vi "PCO_Grab_Save.vi"(7 "# of frames":u16, 8 "entrée d'erreur (pas d'erreur)":errorcluster, 9 "Message Data":variant, 11 "Camera en entrée":refnum<class "Camera.lvclass">) -> (0 "sortie d'erreur":errorcluster, 1 "meta_data_list":T1(array[cluster]), 2 "Raw data (U16)":u16[][][](array[numeric]), 3 "Camera en sortie":refnum<class "Camera.lvclass">)   [LabVIEW 2026]
uses:
  <instrlib>/PCO_SDK/File Group 0/vi.lib/Excelitas PCO GmbH/pco.labview/camera/Camera.lvclass
  Controls/PCO_Config.ctl
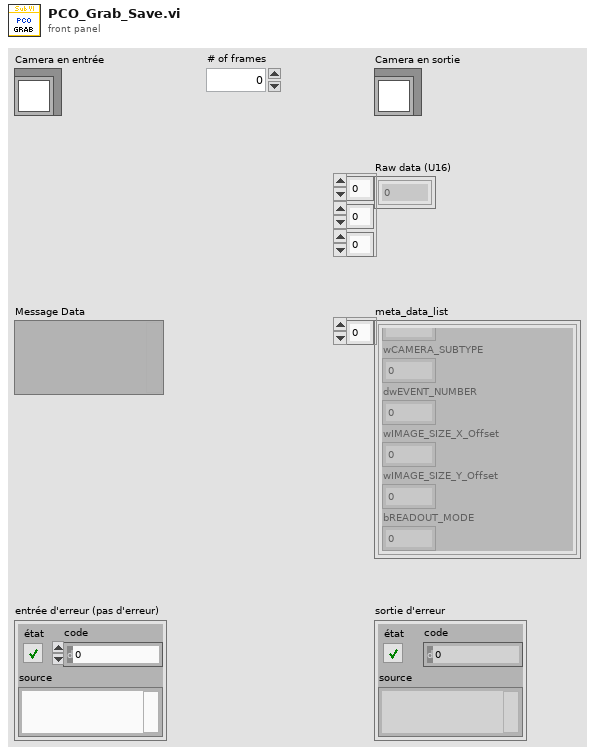
[diagram p1: front panel]
types:
  T1 = cluster{"wVersion":u16, "dwIMAGE_COUNTER":u32, "dwIMAGE_TIME_US":u32, "lvTimestamp":timestamp, "bIMAGE_TIME_STATUS":u8, "wEXPOSURE_TIME_BASE":u16, "dwEXPOSURE_TIME":u32, "dwFRAMERATE_MILLIHZ":u32, "sSENSOR_TEMPERATURE":i16, "wIMAGE_SIZE_X":u16, "wIMAGE_SIZE_Y":u16, "bBINNING_X":u8, "bBINNING_Y":u8, "dwSENSOR_READOUT_FREQUENCY":u32, "wSENSOR_CONV_FACTOR":u16, "dwCAMERA_SERIAL_NO":u32, "wCAMERA_TYPE":u16, "bBIT_RESOLUTION":u8, "bSYNC_STATUS":u8, "wDARK_OFFSET":u16, "bTRIGGER_MODE":u8, "bDOUBLE_IMAGE_MODE":u8, "bCAMERA_SYNC_MODE":u8, "bIMAGE_TYPE":u8, "wCOLOR_PATTERN":u16, "wCAMERA_SUBTYPE":u16, "dwEVENT_NUMBER":u32, "wIMAGE_SIZE_X_Offset":u16, "wIMAGE_SIZE_Y_Offset":u16, "bREADOUT_MODE":u8}[]
  T2 = enum16{"Undefined", "Mono8", "Mono16", "BGRA8", "RGBA8", "BGRA16", "RGBA16", "CompressedMono8"}
  T3 = typedef "PCO_Config.ctl" = cluster{"Exposure time (s)":dbl, "TriggerMode":u16, "ROI X0":u16, "ROI Y0":u16, "ROI X1":u16, "ROI Y1":u16, "Binning":u8}
  T4 = enum16{"sequence", "sequence non blocking", "ring buffer", "fifo", "sequence_dpcore", "sequence_non_blocking_dpcore", "ring_buffer_dpcore", "fifo_dpcore", "tif", "multitif", "pcoraw", "b16", "dicom", "multidicom", "camram_ring", "camram_segment"}
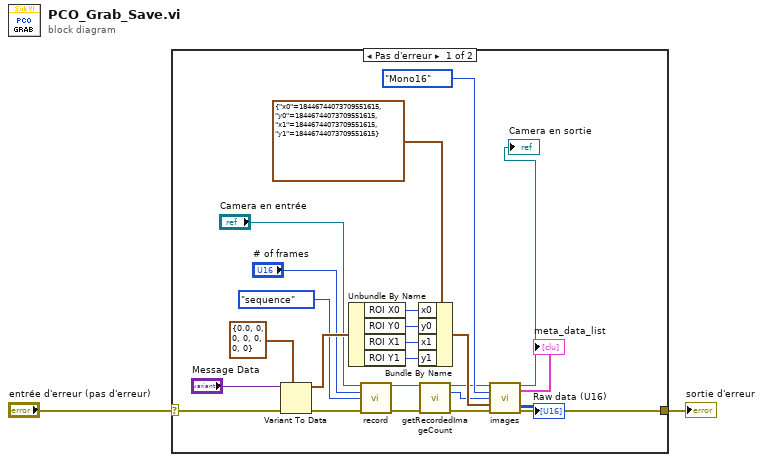
[diagram p0: block diagram]
diagram:
  n1 = case shown="Pas d'erreur" "entrée d'erreur (pas d'erreur)" {
    selector: "entrée d'erreur (pas d'erreur)" -> [w6 w27]
    tunnel: [w5 w27] -> w2
    frame No Error {
      n2 = Variant To Data(error in=w6, type=T3 {"Exposure time (s)"=0.0, "TriggerMode"=0, "ROI X0"=0, "ROI Y0"=0, "ROI X1"=0, "ROI Y1"=0, "Binning"=0} ("PCO_Config"), Variant="Message Data") -> (data=w20:T3, error out=w17:errorcluster)
      n3 = Unbundle By Name(w20) -> ("ROI X0"=w24:u16, "ROI Y0"=w23:u16, "ROI X1"=w22:u16, "ROI Y1"=w21:u16)
      n4 = call-dynamic "record.vi"("Camera in"="Camera en entrée", "num_images"="# of frames", "record_mode"=T4."sequence", "error in (no error)"=w17) -> ("Camera out"=w8:refnum<class "Camera.lvclass">, "error out"=w9:errorcluster)  [unwired: 10 in]
      n5 = Bundle By Name(cluster=cluster{"x0":u64, "y0":u64, "x1":u64, "y1":u64} {"x0"=18446744073709551615, "y0"=18446744073709551615, "x1"=18446744073709551615, "y1"=18446744073709551615} ("roi"), "x0"=w24, "y0"=w23, "x1"=w22, "y1"=w21) -> (w25:cluster{"x0":u64, "y0":u64, "x1":u64, "y1":u64})
      n6 = call-dynamic "getRecordedImageCount.vi"("Camera in"=w8, "error in (no error)"=w9) -> ("Camera out"=w10:refnum<class "Camera.lvclass">, "recorded_image_count"=w13:u32, "error out"=w11:errorcluster)  [unwired: 11 in]
      n7 = call-dynamic "images.vi"("Camera in"=w10, "data_format"=T2."Mono16", "image_count"=w13, "roi"=w25, "error in (no error)"=w11) -> ("meta_data_list"=→"meta_data_list":T1, "Camera out"=→"Camera en sortie":refnum<class "Camera.lvclass">, "raw_image_list (U16)"=→"Raw data (U16)":u16[][][], "error out"=w5:errorcluster)  [unwired: 2 in, 5 out]
    }
    frame Error {
    }
  }
  "sortie d'erreur" <- w2
